vi "Flatten Macro into Table.vi"() -> ()   [LabVIEW 2014]
uses:
  <vilib>/Utility/file.llb/Read From Spreadsheet File (string).vi
  <vilib>/Utility/file.llb/Write To Spreadsheet File (string).vi
  <vilib>/regexp/Match Regular Expression.xnode
panel:
  out "appended array":string[][](array[string])
  out "subarray":string[](array[string])
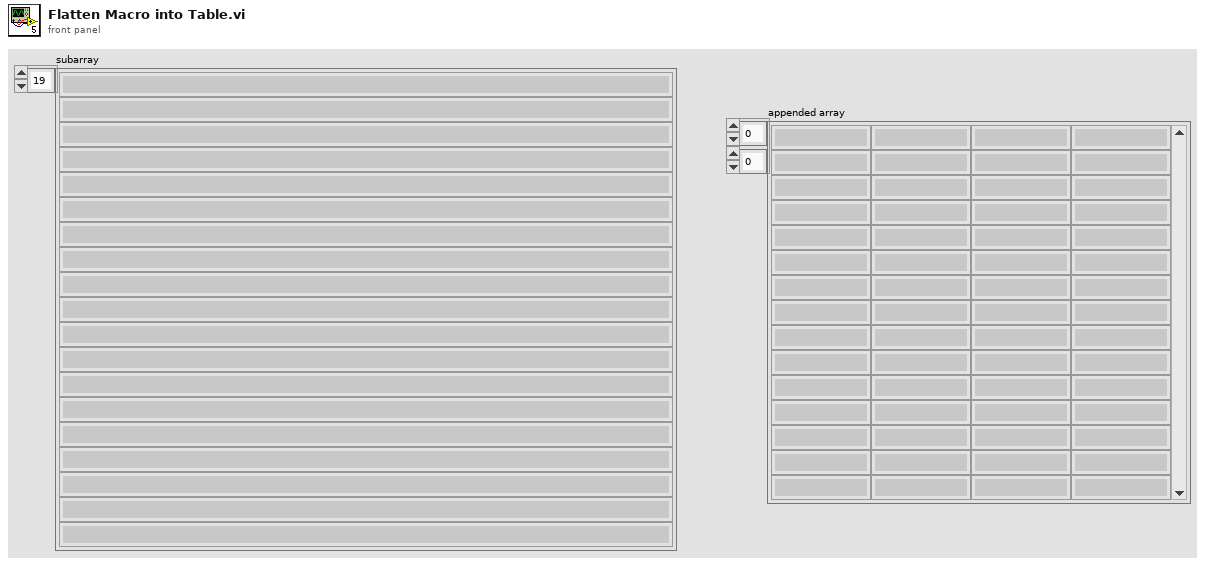
[diagram p1: front panel]
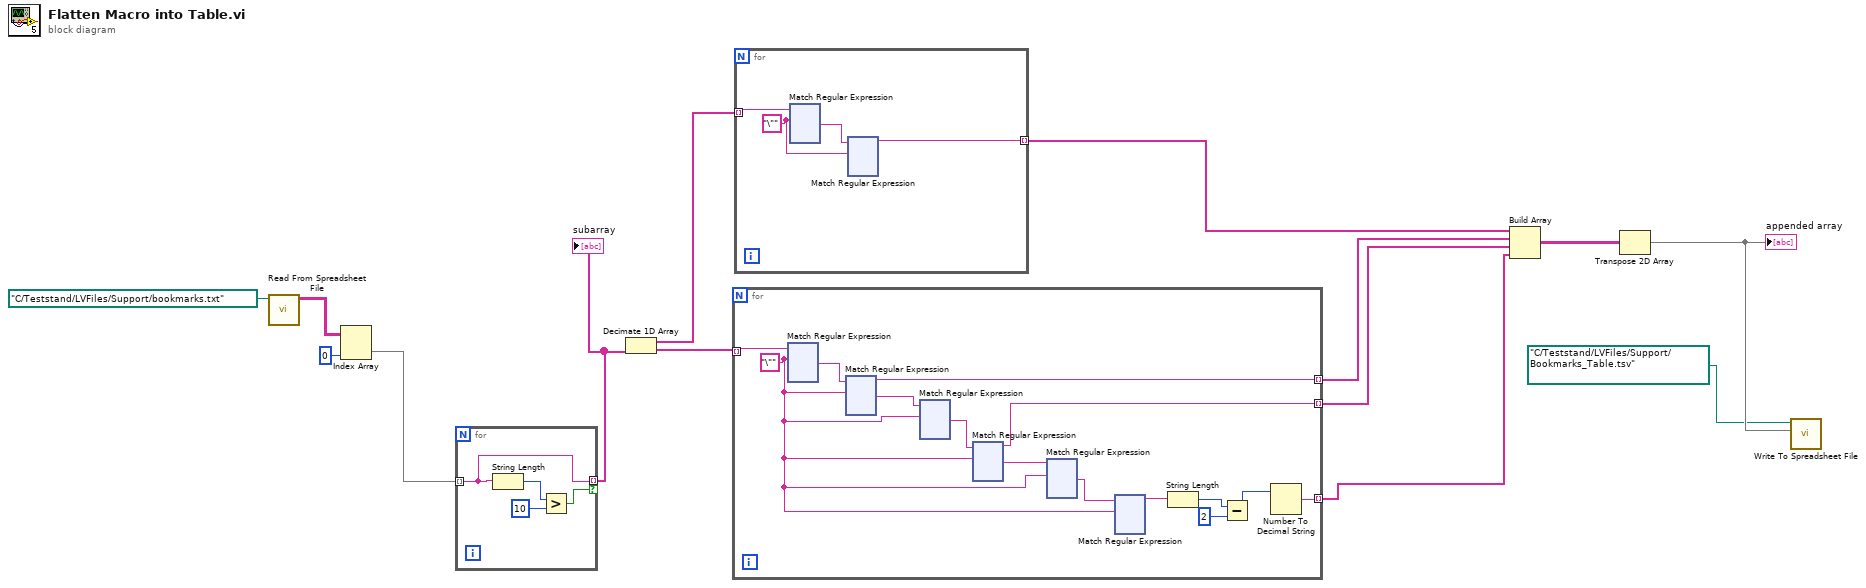
[diagram p0: block diagram]
diagram:
  n1 = call-poly <vilib>:"Read From Spreadsheet File.vi"("file path (dialog if empty)"=path "C:/Teststand/LVFiles/Support/bookmarks.txt") -> ("all rows"=w13:string[][])  [unwired: 6 in, 4 out]
  n2 = Index Array(array=w13, index (col)=0 ("disabled index (col)")) -> (element=w4:string[])  [unwired: 1 in]
  n3 = for {
    tunnel: w4 -> [w18] mode=indexing
    tunnel: [w18] -> w3 mode=indexing if=w15
    n4 = String Length(string=w18) -> (length=w17:i32)
    n5 = Greater?(x=w17, y=10) -> (0:w15:bool)
  }
  "subarray" <- w3
  n6 = Decimate 1D Array(w3) -> (w10:string[], w11:string[])
  n7 = for {
    tunnel: w11 -> [w32] mode=indexing
    tunnel: [w30] -> w8 mode=indexing
    tunnel: [w27] -> w7 mode=indexing
    tunnel: [w22] -> w6 mode=indexing
    w24 = "\"" ("search string/char (-)")
    n8 = xnode "Match Regular Expression"("input string"=w32, "regular expression"=w24) -> ("after match"=w31:string)  [unwired: 4 in, 4 out]
    n9 = xnode "Match Regular Expression"("input string"=w31, "regular expression"=w24) -> ("before match"=w30:string, "after match"=w29:string)  [unwired: 4 in, 3 out]
    n10 = xnode "Match Regular Expression"("input string"=w29, "regular expression"=w24) -> ("after match"=w28:string)  [unwired: 4 in, 4 out]
    n11 = xnode "Match Regular Expression"("input string"=w28, "regular expression"=w24) -> ("before match"=w27:string, "after match"=w26:string)  [unwired: 4 in, 3 out]
    n12 = xnode "Match Regular Expression"("input string"=w26, "regular expression"=w24) -> ("after match"=w25:string)  [unwired: 4 in, 4 out]
    n13 = xnode "Match Regular Expression"("input string"=w25, "regular expression"=w24) -> ("before match"=w23:string)  [unwired: 4 in, 4 out]
    n14 = String Length(string=w23) -> (length=w20:i32)
    n15 = Subtract(x=w20, y=2) -> (x-y=w21:i32)
    n16 = Number To Decimal String(number=w21) -> (decimal integer string=w22:string)  [unwired: 1 in]
  }
  n17 = for {
    tunnel: w10 -> [w720] mode=indexing
    tunnel: [w717] -> w9 mode=indexing
    w718 = "\"" ("search string/char (-)")
    n18 = xnode "Match Regular Expression"("input string"=w720, "regular expression"=w718) -> ("after match"=w719:string)  [unwired: 4 in, 4 out]
    n19 = xnode "Match Regular Expression"("input string"=w719, "regular expression"=w718) -> ("before match"=w717:string)  [unwired: 4 in, 4 out]
  }
  n20 = Build Array(w9, w8, w7, w6) -> (w5:string[][])
  n21 = Transpose 2D Array(2D array=w5) -> (transposed array=w2:string[][])
  "appended array" <- w2
  n22 = call-poly <vilib>:"Write To Spreadsheet File.vi"("2D data"=w2, "file path (dialog if empty)"=path "C:/Teststand/LVFiles/Support/Bookmarks_Table.tsv") -> ()  [unwired: 6 in, 1 out]
